vi "clean_directory.vi"(8 "error in":errorcluster, 11 "DirReport":path=path "L:/Documentos/00 SERVIÇOS/Tensão residual/Olapa 10-2017/RelatóriosOlapa/Teste" caption="Pasta do relatório") -> (0 "error out":errorcluster, 3 "DirOut":path=path "L:/Documentos/00 SERVIÇOS/Tensão residual/Olapa 10-2017/RelatóriosOlapa/Teste" caption="Pasta do relatório")   [LabVIEW 2016]
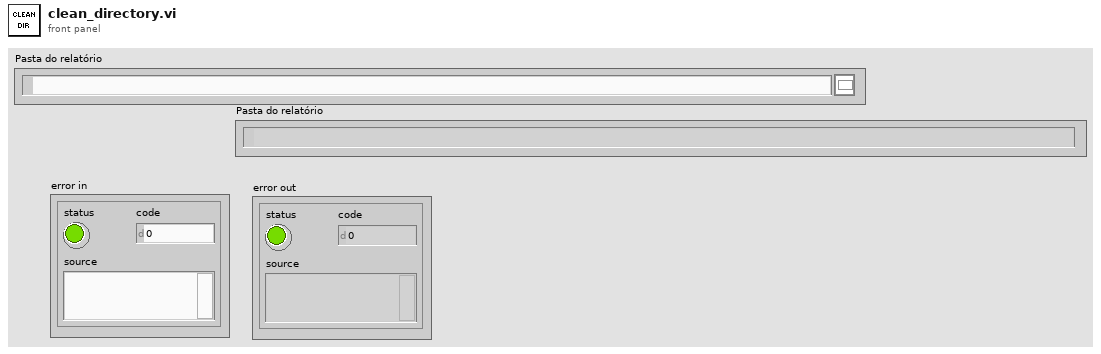
[diagram p1: front panel]
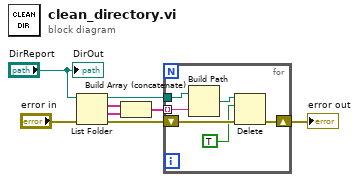
[diagram p0: block diagram]
diagram:
  n1 = List Folder(path="DirReport", error in="error in") -> (path out=w4:path, filenames=w7:string[], folder names=w6:string[], error out=w3:errorcluster)  [unwired: 2 in]
  n2 = Build Array (concatenate)(w7, w6) -> (w5:string[])
  n3 = for {
    tunnel: w5 -> [w14] mode=indexing
    tunnel: w4 -> [w13]
    shift-right: [w10] -> w2
    shift-left: w3 -> [w11]
    n4 = Build Path(base path=w13, name or relative path=w14) -> (appended path=w12:path)
    n5 = Delete(path (use dialog)=w12, entire hierarchy (F)=TRUE, error in=w11) -> (error out=w10:errorcluster)  [unwired: 2 in, 2 out]
  }
  "error out" <- w2
  "DirOut" <- "DirReport"
